vi "Tx Bool flag set true_USRP1_demoinfocom.vi"(3 "error in (no error)":errorcluster) -> (10 "error out":errorcluster)   [LabVIEW 2021]
uses:
  system stop.vi
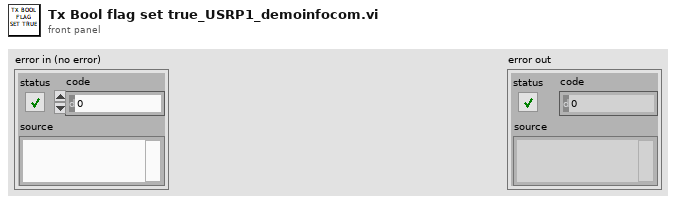
[diagram p1: front panel]
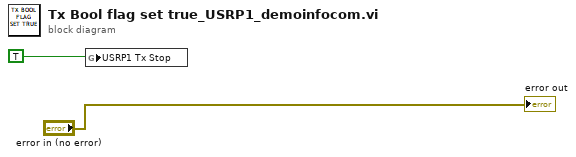
[diagram p0: block diagram]
diagram:
  n1 = global write "system stop.vi" "USRP1 Tx Stop"(TRUE) -> ()
  "error out" <- "error in (no error)"
